vi "ReadDataGen.vi"(0 "path":path, 11 "error in (no error)":errorcluster) -> (4 "Initial Info":string, 6 "ScanHdr":string, 8 "Scan Data":dbl[][](array[numeric]), 15 "error out":errorcluster)   [LabVIEW 2010]
panel:
  out "Date":string
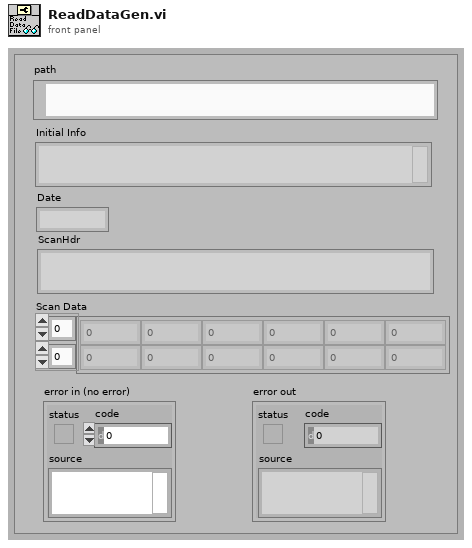
[diagram p1: front panel]
types:
  T1 = enum16{"open", "open or create", "create or replace", "create", "open (read only)"}
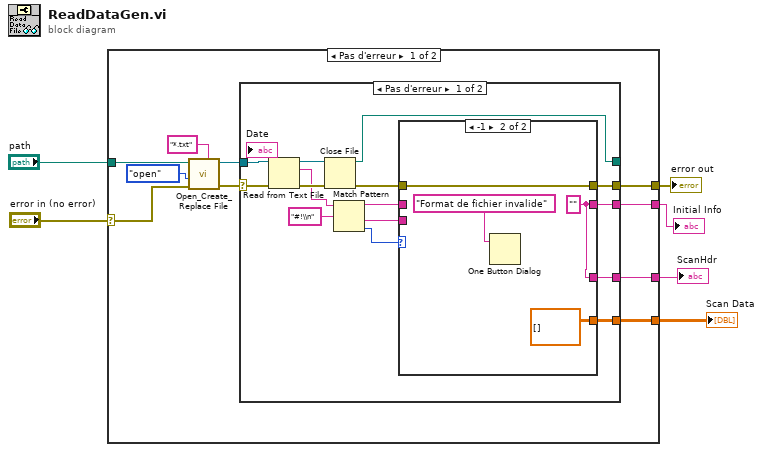
[diagram p0: block diagram]
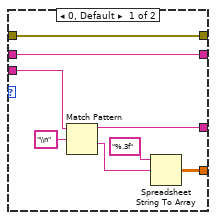
[diagram p2: hidden frame]
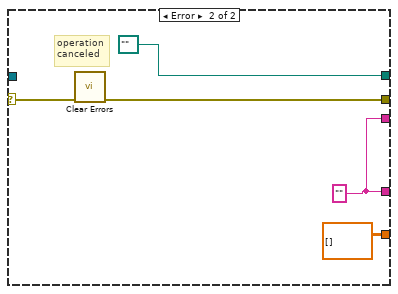
[diagram p3: hidden frame]
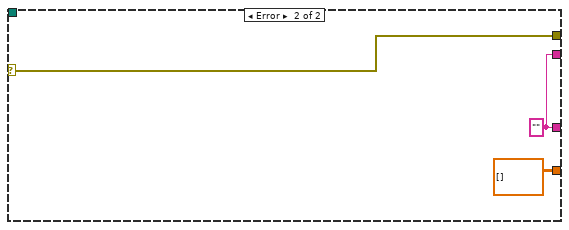
[diagram p4: hidden frame]
diagram:
  n1 = case shown="Pas d'erreur" "error in (no error)" {
    selector: "error in (no error)" -> [w14 w51]
    tunnel: [w10 w51] -> w5
    tunnel: "path" -> [w15 _]
    tunnel: [w9 w50] -> w2
    tunnel: [w8 w50] -> w1
    tunnel: [w7 dbl[][] []] -> w3
    frame No Error {
      n2 = call <vilib>:"Open_Create_Replace File.vi"("pattern"="*.txt", "error in (no error)"=w14, "function (open:0)"=T1."open", "file path"=w15) -> ("error out"=w13:errorcluster, "refnum"=w12:refnum<file>)  [unwired: 4 in, 2 out]
      n3 = case shown="Pas d'erreur" w13 {
        selector: w13 -> [w30 w48]
        tunnel: [w17 w47] -> w10
        tunnel: [w19 path "" ("path")] -> _
        tunnel: w12 -> [w31 _]
        tunnel: [w24 w45] -> w8
        tunnel: [w20 w45] -> w9
        tunnel: [w25 dbl[][] []] -> w7
        frame No Error {
          n4 = Read from Text File(file (use dialog)=w31, error in=w30) -> (refnum out=w29:refnum<file>, text=w26:string, error out=w28:errorcluster)  [unwired: 2 in, 1 out]
          n5 = Close File(refnum=w29, error in=w28) -> (path=w19:path, error out=w18:errorcluster)
          n6 = Match Pattern(string=w26, regular expression="#!\\n" ("expression régulière")) -> (before substring=w21:string, after substring=w23:string, offset past match=w22:i32)  [unwired: 1 in, 1 out]
          n7 = case shown="-1" w22 {
            tunnel: [w39 dbl[][] []] -> w25
            tunnel: [w38 w41] -> w24
            tunnel: w23 -> [w35 _]
            tunnel: w21 -> [w32 _]
            tunnel: [w32 w41] -> w20
            tunnel: w18 -> [w33 w43]
            tunnel: [w33 w43] -> w17
            frame 0, Default {
              n8 = Match Pattern(string=w35, regular expression="\\n" ("expression régulière")) -> (before substring=w38:string, after substring=w37:string)  [unwired: 1 in, 2 out]
              n9 = Spreadsheet String To Array(format string="%.3f" ("chaîne de format"), spreadsheet string=w37) -> (array=w39:dbl[][])  [unwired: 2 in]
            }
            frame -1 {
              w41 = ""
              n10 = One Button Dialog(message="Format de fichier invalide") -> ()  [unwired: 1 in, 1 out]
            }
          }
        }
        frame Error {
          w45 = ""
          # "operation\ncanceled"
          n11 = call <vilib>:"Clear Errors.vi"("error in (no error)"=w48) -> ("error out"=w47:errorcluster)  [unwired: 6 in]
        }
      }
    }
    frame Error {
      w50 = ""
    }
  }
  "error out" <- w5
  "ScanHdr" <- w1
  "Scan Data" <- w3
  "Initial Info" <- w2
